vi "OAT Multistage Interpolator Decimator Design.vi"(7 "alias free":bool, 9 "A stop [dB]":dbl=72.0 format="%.2f", 10 "bandwidth (auto)":cluster{"passband":dbl, "stopband":dbl} {"stopband" format="%.2f"; "passband" format="%.2f"}, 11 "interpolation/decimation factor":i32=2) -> (0 "error out":errorcluster, 1 "filter":T1[](array[typedef]) {"coefficients" format="%.2f"})   [LabVIEW 2017, in "SoundVib_Resampling.lvlib"]
doc: "Design a multistage interpolation/decimation filter."
uses:
  <vilib>/addons/Sound and Vibration/Order Analysis/Resample Order Tracking/SoundVib_Resampling.lvlib
  <vilib>/addons/_NISVFA/_Shared subVIs/Controls/OAT Decimation Filter.ctl
panel:
  in  "x < y?":bool
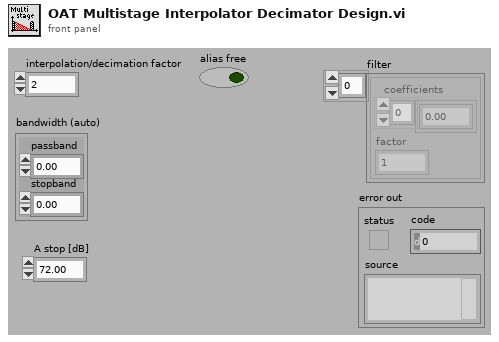
[diagram p1: front panel]
types:
  T1 = typedef "OAT Decimation Filter.ctl" = cluster{"coefficients":dbl[], "factor":i32}
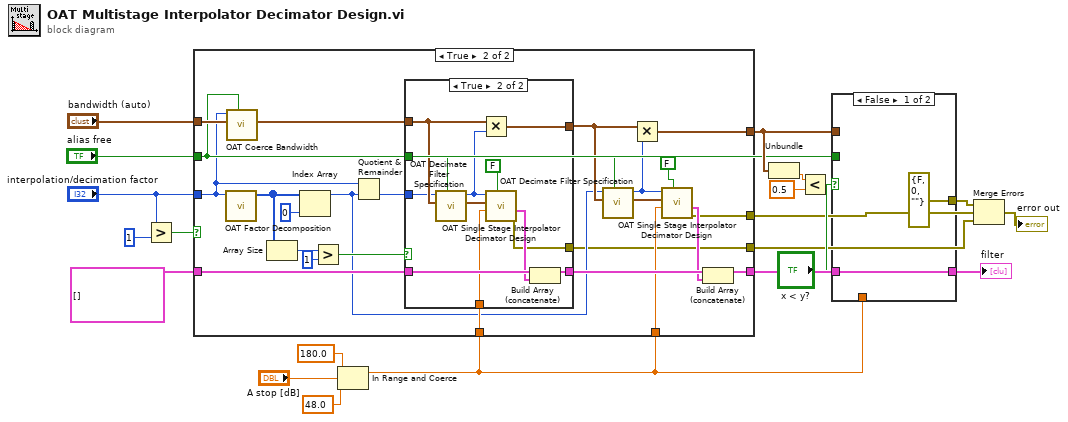
[diagram p0: block diagram]
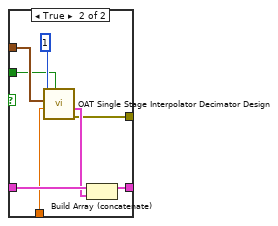
[diagram p2: hidden frame]
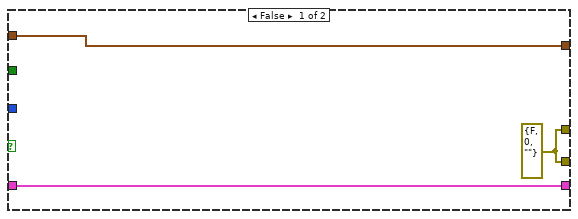
[diagram p3: hidden frame]
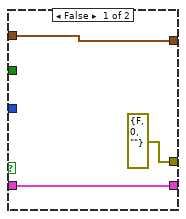
[diagram p4: hidden frame]
diagram:
  n1 = Greater?(x="interpolation/decimation factor", y=1) -> (0:w19:bool)
  n2 = In Range and Coerce(upper limit=180.0, x="A stop [dB]", lower limit=48.0) -> (coerced(x)=w8:dbl)  [unwired: 1 out]
  n3 = case shown="True" w19 {
    tunnel: "interpolation/decimation factor" -> [_ w32]
    tunnel: "bandwidth (auto)" -> [w23 w34]
    tunnel: w8 -> [_ w29]
    tunnel: [w23 w40] -> w11
    tunnel: w8 -> [_ w39]
    tunnel: T1[] [] ("multistage decimator") -> [w22 w38]
    tunnel: [w22 w35] -> w13
    tunnel: "alias free" -> [_ w27]
    tunnel: [w21 w25] -> w2
    tunnel: [w21 w24] -> w3
    frame False {
      w21 = errorcluster {"status"=FALSE, "code"=0, "source"=""} ("error out")
    }
    frame True {
      n4 = call <vilib>:"OAT Factor Decomposition.vi"("number"=w32) -> ("factors"=w47:i32[])  [unwired: 3 in, 3 out]
      n5 = call <vilib>:"OAT Coerce Bandwidth.vi"("alias free"=w27, "bandwidth (auto)"=w34, "interpolation/decimation factor"=w32) -> ("bandwidth out"=w33:cluster{"passband":dbl, "stopband":dbl})  [unwired: 8 in]
      n6 = Array Size(array=w47) -> (size(s)=w46:i32)
      n7 = Index Array(array=w47, index=0 ("Index")) -> (element=w26:i32)
      n8 = Greater?(x=w46, y=1) -> (0:w43:bool)
      n9 = Quotient & Remainder(x=w32, y=w26) -> (floor(x/y)=w31:i32)  [unwired: 1 out]
      n10 = case shown="True" w43 {
        tunnel: w33 -> [w50 w61]
        tunnel: w31 -> [_ w60]
        tunnel: [w50 w59] -> w41
        tunnel: w39 -> [_ w54]
        tunnel: w38 -> [w49 w58]
        tunnel: [w49 w56] -> w37
        tunnel: w27 -> [_ w52]
        tunnel: [errorcluster {"status"=FALSE, "code"=0, "source"=""} ("error out") w51] -> w25
        frame False {
        }
        frame True {
          n11 = call <vilib>:"OAT Decimate Filter Specification.vi"("alias free"=w52, "bandwidth"=w61, "interpolation/decimation factor"=w60) -> ("bandwidth"=w55:cluster{"passband":dbl, "stopband":dbl}, "current factor"=w62:i32)  [unwired: 7 in]
          n12 = Multiply(x=w61, y=w62) -> (x*y=w59:cluster{"passband":dbl, "stopband":dbl})
          n13 = call <vilib>:"OAT Single Stage Interpolator Decimator Design.vi"("alias free"=FALSE, "A stop [dB]"=w54, "bandwidth (auto)"=w55, "interpolation/decimation factor"=w62) -> ("error out"=w51:errorcluster, "filter"=w57:T1)  [unwired: 6 in]
          n14 = Build Array (concatenate)(w58, w57) -> (w56:T1[])
        }
      }
      n15 = call <vilib>:"OAT Decimate Filter Specification.vi"("alias free"=w27, "bandwidth"=w41, "interpolation/decimation factor"=w26) -> ("bandwidth"=w42:cluster{"passband":dbl, "stopband":dbl}, "current factor"=w30:i32)  [unwired: 7 in]
      n16 = Multiply(x=w41, y=w30) -> (x*y=w40:cluster{"passband":dbl, "stopband":dbl})
      n17 = call <vilib>:"OAT Single Stage Interpolator Decimator Design.vi"("alias free"=FALSE, "A stop [dB]"=w29, "bandwidth (auto)"=w42, "interpolation/decimation factor"=w30) -> ("error out"=w24:errorcluster, "filter"=w36:T1)  [unwired: 6 in]
      n18 = Build Array (concatenate)(w37, w36) -> (w35:T1[])
    }
  }
  n19 = Unbundle(w11) -> ("stopband"=w16:dbl)  [unwired: 1 out]
  n20 = Less?(x=w16, y=0.5) -> ()  [unwired: 1 out]
  n21 = case shown="False" "x < y?" {
    tunnel: w8 -> [_ w67]
    tunnel: w13 -> [w64 w71]
    tunnel: [w64 w69] -> w12
    tunnel: w11 -> [_ w68]
    tunnel: "alias free" -> [_ w66]
    tunnel: [errorcluster {"status"=FALSE, "code"=0, "source"=""} ("error out") w65] -> w4
    frame False {
    }
    frame True {
      n22 = call <vilib>:"OAT Single Stage Interpolator Decimator Design.vi"("alias free"=w66, "A stop [dB]"=w67, "bandwidth (auto)"=w68, "interpolation/decimation factor"=1 ("interpolate factor")) -> ("error out"=w65:errorcluster, "filter"=w70:T1)  [unwired: 6 in]
      n23 = Build Array (concatenate)(w71, w70) -> (w69:T1[])
    }
  }
  "filter" <- w12
  n24 = Merge Errors(w4, w3, w2) -> (→"error out":errorcluster)
